vi "Configure Sequence Parameters.vi"(0 "VISA resource name":refnum<visa-resource-name>, 1 "Step Voltage (1.000)":dbl=1.0 format="%.3g", 2 "Step Number (1)":dbl=1.0 min=1.0 max=10.0 step=1.0 format="%#.0p", 5 "Step Current (1.000)":dbl=1.0 format="%.3g", 7 "Step Width (1)":dbl=1.0 min=0.001 max=65.535 step=0.001 format="%.3f", 9 "Step Slope (1)":dbl=1.0 min=0.0010000000474974513 max=65.53500366210938 step=0.0010000000474974513 format="%.3f", 11 "error in (no error)":errorcluster) -> (4 "VISA resource name out":refnum<visa-resource-name>, 15 "error out":errorcluster)   [LabVIEW 2020, in "BK Precision 911X Series.lvlib"]
doc: "Configures the step parameters of a selected sequence. Run this vi after running <b>Configure Sequence.vi</b>. The steps configured with this vi should match the steps that are active, which are configured within <b>Configure Sequence.vi</b> with the parameter <b>Active Steps</b>. If a step is not configured and is active, it will have a default value from factory settings.\n\n<b>Note: When all steps parameters are configured, run the Save Sequence.vi to save all configurations into the memory of the instrument. Sequence function is not supported for model 9117.</b>"
uses:
  BK Precision 911X Series.lvlib
panel:
  # "s"
  # "s"
  # "A"
  # "V"
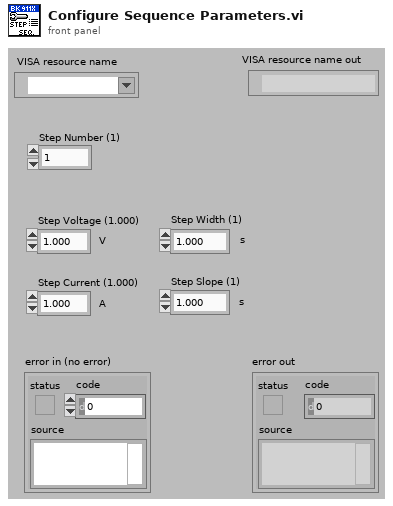
[diagram p1: front panel]
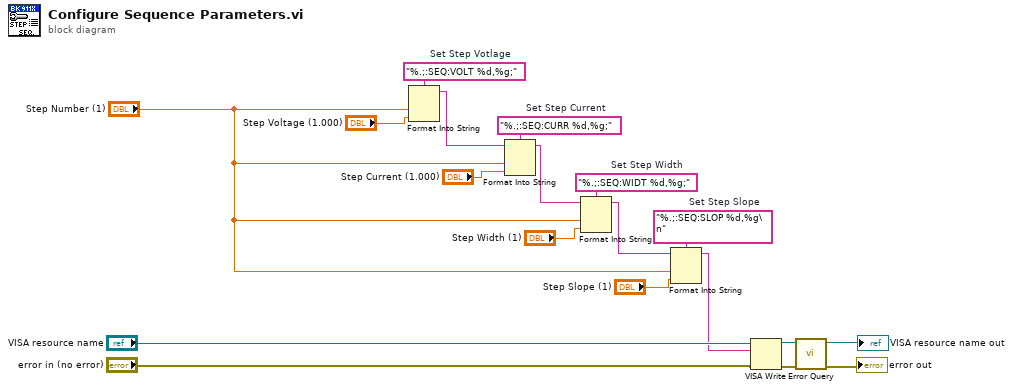
[diagram p0: block diagram]
diagram:
  w11 = "%.;:SEQ:VOLT %d,%g;"  # Set Step Votlage
  w12 = "%.;:SEQ:CURR %d,%g;"  # Set Step Current
  w17 = "%.;:SEQ:SLOP %d,%g\n"  # Set Step Slope
  w19 = "%.;:SEQ:WIDT %d,%g;"  # Set Step Width
  n1 = Format Into String(format string=w11, "Step Number (1)", "Step Voltage (1.000)") -> (resulting string=w10:string)  [unwired: 2 in, 1 out]
  n2 = Format Into String(format string=w12, initial string=w10, "Step Number (1)", "Step Current (1.000)") -> (resulting string=w9:string)  [unwired: 1 in, 1 out]
  n3 = Format Into String(format string=w19, initial string=w9, "Step Number (1)", "Step Width (1)") -> (resulting string=w18:string)  [unwired: 1 in, 1 out]
  n4 = Format Into String(format string=w17, initial string=w18, "Step Number (1)", "Step Slope (1)") -> (resulting string=w3:string)  [unwired: 1 in, 1 out]
  n5 = VISA Write(VISA resource name="VISA resource name", write buffer=w3, error in (no error)="error in (no error)") -> (VISA resource name out=w16:refnum<visa-resource-name>, error out=w15:errorcluster)  [unwired: 1 out]
  n6 = call "Error Query.vi"("error in (no error)"=w15, "VISA resource name"=w16) -> ("error out"=→"error out":errorcluster, "VISA resource name out"=→"VISA resource name out":refnum<visa-resource-name>)  [unwired: 6 in, 2 out]
